vi "Inplace SubArray Replace.vi"() -> ()   [LabVIEW 2016]
panel:
  out "Resultant Data":i32[](array[numeric])
  in  "Start Index":i32
  in  "Replacement Data":i32[](array[numeric])
  in  "Source Data":i32[](array[numeric])=[1, 1, 1, 1, 1, 1, 1, 1, 1, 1]
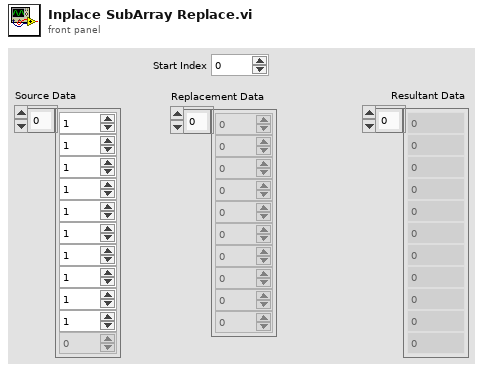
[diagram p1: front panel]
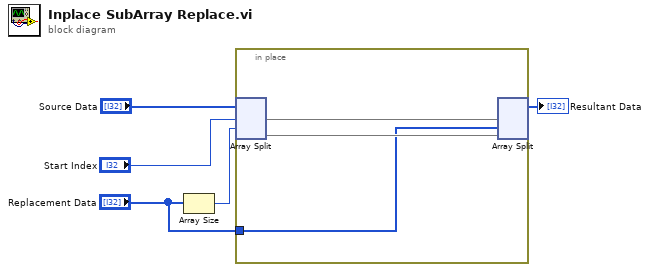
[diagram p0: block diagram]
diagram:
  n1 = Array Size(array="Replacement Data") -> (size(s)=w4:i32)
  n2 = in-place {
    in-place-border: "Replacement Data" -> [w6]
    n3 = in-place-split #1("Source Data", "Start Index", w4) -> (w8:i32[], w7:i32[])  [unwired: 1 out]
    n4 = in-place-split #1(w8, w6, w7) -> (→"Resultant Data":i32[])  [unwired: 2 out]
  }
